vi "Render.vi"(8 "error in (no error)":errorcluster, 10 "String in":string, 11 "Url in":refnum<class "Url.lvclass">) -> (0 "error out":errorcluster, 2 "String out":string, 3 "Url out":refnum<class "Url.lvclass">)   [LabVIEW 2021, in "Markdown.lvlib" / "Url.lvclass"]
uses:
  Url.lvclass
  C:/GitHub/Markdown/src/Markdown/Markdown.lvclass
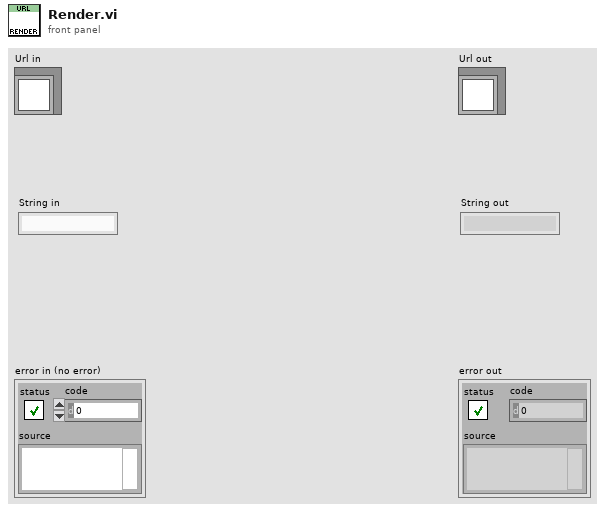
[diagram p1: front panel]
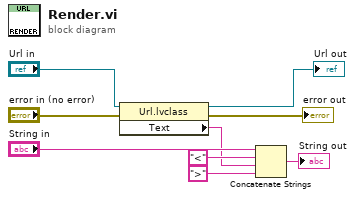
[diagram p0: block diagram]
diagram:
  n1 = property class="Url.lvclass"(reference="Url in", error in="error in (no error)") -> (reference out=→"Url out":refnum<class "Url.lvclass">, error out=→"error out":errorcluster, "Text"=w2:string)
  n2 = Concatenate Strings("String in", "<" ("string"), w2, ">" ("string")) -> (→"String out":string)
